vi "uA_daq_capture_small_curr_waveform.vi"(9 "Sample rate":dbl, 10 "CrsrList":T1, 11 "Waveform_main":waveform(sgl)) -> (3 "Numeric":sgl)   [LabVIEW 2015]
uses:
  <vilib>/Utility/miscctls.llb/LVCursorListTypeDef.ctl
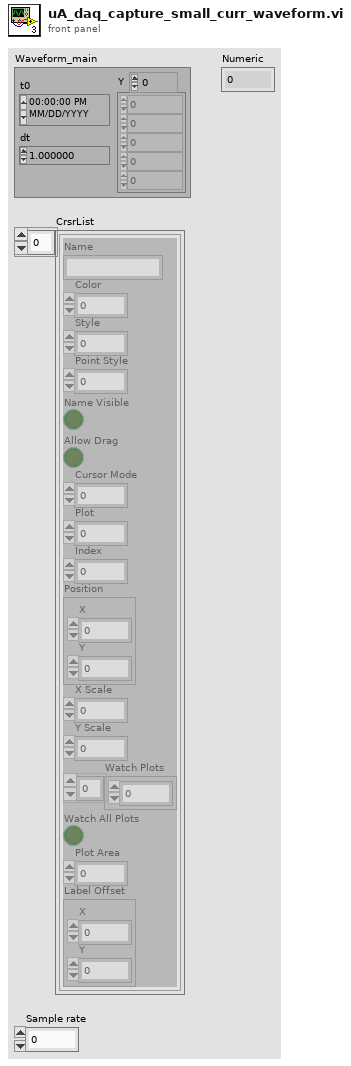
[diagram p1: front panel]
types:
  T1 = typedef "LVCursorListTypeDef.ctl" = cluster{"Name":string, "Color":u32, "Style":u8, "Point Style":u8, "Name Visible":bool, "Allow Drag":bool, "Cursor Mode":u32, "Plot":i32, "Index":i32, "Position":cluster{"X":dbl, "Y":dbl}, "X Scale":u32, "Y Scale":u32, "Watch Plots":i32[], "Watch All Plots":bool, "Plot Area":i32, "Label Offset":cluster{"X":dbl, "Y":dbl}}[]
  T2 = cluster{"Name":string, "Color":u32, "Style":u8, "Point Style":u8, "Name Visible":bool, "Allow Drag":bool, "Cursor Mode":u32, "Plot":i32, "Index":i32, "Position":cluster{"X":dbl, "Y":dbl}, "X Scale":u32, "Y Scale":u32, "Watch Plots":i32[], "Watch All Plots":bool, "Plot Area":i32, "Label Offset":cluster{"X":dbl, "Y":dbl}}
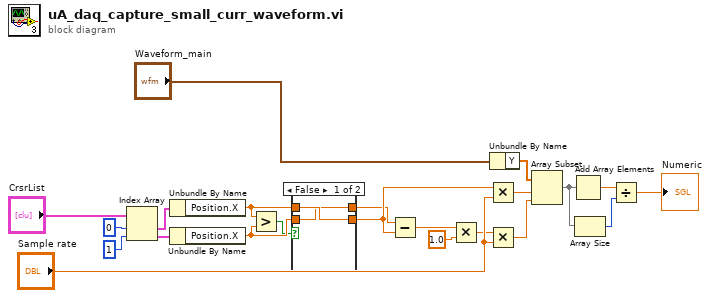
[diagram p0: block diagram]
diagram:
  n1 = Index Array(array="CrsrList", index #1=0 ("index"), index #2=1 ("index")) -> (element #1=w9:T2, element #2=w13:T2)
  n2 = Unbundle By Name(w9) -> ("Position.X"=w16:dbl)
  n3 = Unbundle By Name(w13) -> ("Position.X"=w15:dbl)
  n4 = Greater?(x=w16, y=w15) -> (0:w14:bool)
  n5 = case shown="False" w14 {
    tunnel: w16 -> [w24 w26]
    tunnel: w15 -> [w23 w25]
    tunnel: [w23 w26] -> w17
    tunnel: [w24 w25] -> w18
    frame False {
    }
    frame True {
    }
  }
  n6 = Subtract(x=w17, y=w18) -> (x-y=w19:dbl)
  n7 = Multiply(x=w19, y=1.0) -> (x*y=w8:dbl)
  n8 = Multiply(x=w18, y="Sample rate") -> (x*y=w2:dbl)
  n9 = Multiply(x=w8, y="Sample rate") -> (x*y=w3:dbl)
  n10 = Unbundle By Name("Waveform_main") -> ("Y"=w21:sgl[])
  n11 = Array Subset(array=w21, index=w2, length=w3) -> (w4:sgl[])
  n12 = Add Array Elements(numeric array=w4) -> (sum=w5:sgl)
  n13 = Array Size(array=w4) -> (size(s)=w6:i32)
  n14 = Divide(x=w5, y=w6) -> (x/y=→"Numeric":sgl)
